vi "Update TriggerTillShot.vi"(8 "error in (no error)":errorcluster, 10 "TriggerCounter":i32, 11 "BME_DG_Chnl in":refnum<class "BME_DG_Chnl.lvclass">) -> (0 "error out":errorcluster, 1 "update time":timestamp, 2 "TriggerTillShot":i32, 3 "BME_DG_Chnl out":refnum<class "BME_DG_Chnl.lvclass">)   [LabVIEW 2009, in "BME_DG_Chnl.lvclass"]
uses:
  BME_DG_Chnl.lvclass
  BME_DG_Chnl.lvclass/BME_DG_Chnl.ctl
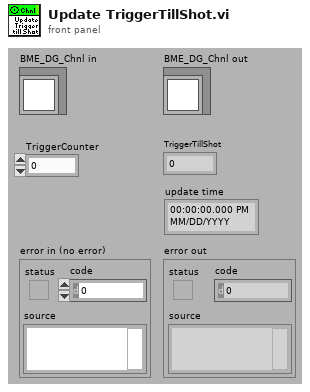
[diagram p1: front panel]
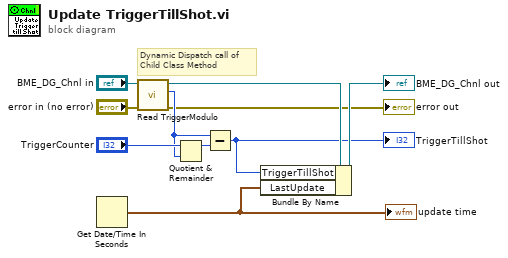
[diagram p0: block diagram]
diagram:
  # "Dynamic Dispatch call of\nChild Class Method"
  n1 = Get Date/Time In Seconds() -> (seconds since 1Jan1904=w7:timestamp)
  "update time" <- w7
  n2 = call-dynamic "Read TriggerModulo.vi"("error in (no error)"="error in (no error)", "BME_DG_Chnl in"="BME_DG_Chnl in") -> ("error out"=→"error out":errorcluster, "TriggerModulo"=w4:i32, "BME_DG_Chnl out"=w5:refnum<class "BME_DG_Chnl.lvclass">)  [unwired: 7 in]
  n3 = Quotient & Remainder(x="TriggerCounter", y=w4) -> (x-y*floor(x/y)=w6:i32)  [unwired: 1 out]
  n4 = Subtract(x=w4, y=w6) -> (x-y=w1:i32)
  "TriggerTillShot" <- w1
  n5 = Bundle By Name(cluster=w5, "TriggerTillShot"=w1, "LastUpdate"=w7) -> (→"BME_DG_Chnl out":refnum<class "BME_DG_Chnl.lvclass">)
